vi "test.vi"() -> ()   [LabVIEW 2018]
panel:
  out "String":string
  in  "XML File Path":path
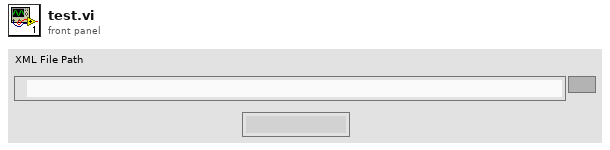
[diagram p1: front panel]
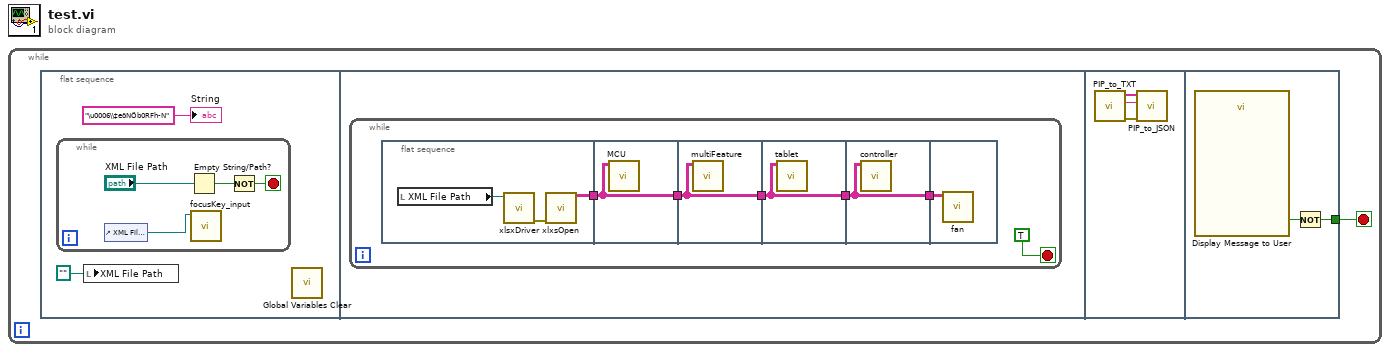
[diagram p0: block diagram]
diagram:
  n1 = while {
    stop <- w1 stop-if-true
    n2 = flat-sequence {
      tunnel: [w25] -> w1
      frame #0 {
        n3 = while {
          stop <- w4 stop-if-true
          n4 = control-ref of="XML File Path"() -> (w7:refnum<vi>)
          n5 = Empty String/Path?(string/path="XML File Path") -> (empty?=w5:bool)
          n6 = call "focusKey_input.vi"("reference"=w7) -> ()  [unwired: 10 in, 1 out]
          n7 = Not(x=w5) -> (.not. x?=w4:bool)
        }
        n8 = local write "XML File Path"(path "") -> ()
        n9 = call "Global Variables Clear.vi"() -> ()  [unwired: 12 in]
        "String" <- "\u0006\\‡eöNÖb0RFh-N"
      }
      frame #1 {
        n10 = while {
          stop <- TRUE stop-if-true
          n11 = flat-sequence {
            tunnel: [w14] -> w12
            tunnel: w12 -> [w17]
            tunnel: [w17] -> w11
            tunnel: w11 -> [w18]
            tunnel: [w18] -> w10
            tunnel: w10 -> [w19]
            tunnel: [w19] -> w9
            tunnel: w9 -> [w20]
            tunnel: [w20] -> w8
            tunnel: w8 -> [w21]
            frame #0 {
              n12 = local read "XML File Path"() -> (w16:path)
              n13 = call "xlsxDriver.vi"("XML File Path"=w16) -> ("error out"=w15:errorcluster)  [unwired: 10 in]
              n14 = call "xlxsOpen.vi"("error in (no error)"=w15) -> ("Shared_strings"=w14:string[][])  [unwired: 10 in, 4 out]
            }
            frame #1 {
              n15 = call "MCU.vi"("Shared_strings"=w17) -> ()  [unwired: 11 in]
            }
            frame #2 {
              n16 = call "multiFeature.vi"("Shared_strings"=w18) -> ()  [unwired: 11 in]
            }
            frame #3 {
              n17 = call "tablet.vi"("Shared_strings"=w19) -> ()  [unwired: 11 in]
            }
            frame #4 {
              n18 = call "controller.vi"("Shared_strings"=w20) -> ()  [unwired: 11 in]
            }
            frame #5 {
              n19 = call "fan.vi"("Shared_strings"=w21) -> ()  [unwired: 11 in]
            }
          }
        }
      }
      frame #2 {
        n20 = call "PIP_to_TXT.vi"() -> ("error out"=w22:errorcluster, "FileName"=w23:string, "PIP_to_JSN"=w24:string[])  [unwired: 9 in]
        n21 = call "PIP_to_JSON.vi"("error in (no error)"=w22, "FileName"=w23, "jsonGen"=w24) -> ()  [unwired: 8 in, 1 out]
      }
      frame #3 {
        n22 = call "Display Message to User"() -> ("YES"=w26:bool)  [unwired: 10 in, 1 out]
        n23 = Not(x=w26) -> (.not. x?=w25:bool)
      }
    }
  }
